vi "ParseSignalConfigCluster.vi"(11 "Signal Channel Config":T1={"Input Mode"=enum."Both Grounded", "Input Connector Shell"=enum."Float", "Input Device"=enum."FET", "Line Rejection Filter"=enum."Off"}) -> (0 "Input Device":bool, 1 "Input Connector Shells":bool, 2 "Input Mode":u16, 3 "Line Frequency\nRejection Filter":u8)   [LabVIEW 2016, in "Instrument.SR7270.lvclass"]
uses:
  Instrument.SR7270.lvclass
  Typedefs/SignalChannelConfig--Cluster.ctl
  Driver/Typedefs/VMODE--enum.ctl
  Driver/SR7270 Drivers.lvclass
  Driver/Typedefs/FLOAT--enum.ctl
  Driver/Typedefs/FET--enum.ctl
  Driver/Typedefs/LF--enum.ctl
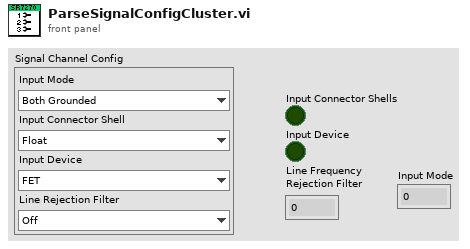
[diagram p1: front panel]
types:
  T1 = typedef "Instrument.SR7270.lvclass/SignalChannelConfig--Cluster.ctl" = cluster{"Input Mode":T2, "Input Connector Shell":T3, "Input Device":T4, "Line Rejection Filter":T5}
  T2 = typedef "SR7270 Drivers.lvclass/VMODE--enum.ctl" = enum16{"Both Grounded", "A input only", "-B input only", "A-B differential"}
  T3 = typedef "SR7270 Drivers.lvclass/FLOAT--enum.ctl" = enum16{"Ground", "Float"}
  T4 = typedef "SR7270 Drivers.lvclass/FET--enum.ctl" = enum16{"Bipolar", "FET"}
  T5 = typedef "SR7270 Drivers.lvclass/LF--enum.ctl" = enum16{"Off", "60 Hz", "120 Hz", "60 & 120 Hz"}
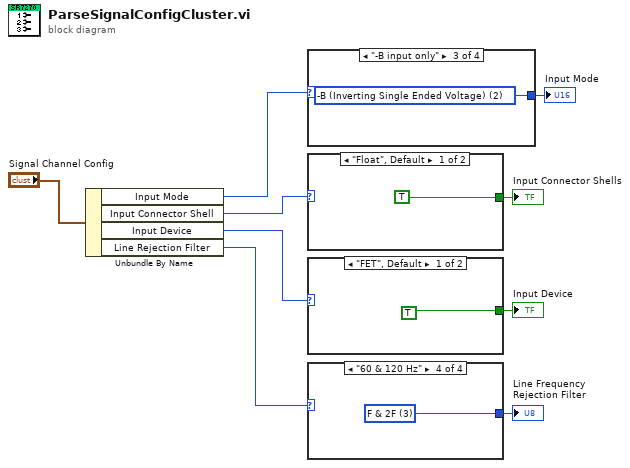
[diagram p0: block diagram]
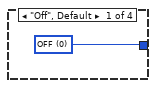
[diagram p2: hidden frame]
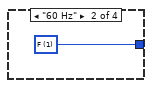
[diagram p3: hidden frame]
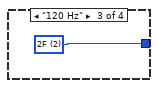
[diagram p4: hidden frame]
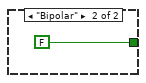
[diagram p5: hidden frame]
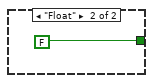
[diagram p6: hidden frame]
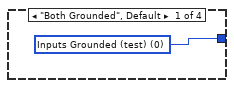
[diagram p7: hidden frame]
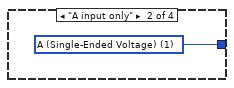
[diagram p8: hidden frame]
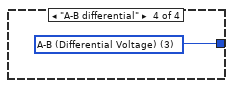
[diagram p9: hidden frame]
diagram:
  n1 = Unbundle By Name("Signal Channel Config") -> ("Input Mode"=w8:T2, "Input Connector Shell"=w7:T3, "Input Device"=w6:T4, "Line Rejection Filter"=w5:T5)
  n2 = case shown="\"-B input only\"" w8 {
    tunnel: [w10 w11 w12 w13] -> w4
    frame "Both Grounded", Default {
      w10 = u16 0 items=["Inputs Grounded (test)", "A (Single-Ended Voltage)", "-B (Inverting Single Ended Voltage)", "A-B (Differential Voltage)"] ("Input Mode")
    }
    frame "A input only" {
      w11 = u16 1 items=["Inputs Grounded (test)", "A (Single-Ended Voltage)", "-B (Inverting Single Ended Voltage)", "A-B (Differential Voltage)"] ("Input Mode")
    }
    frame "-B input only" {
      w12 = u16 2 items=["Inputs Grounded (test)", "A (Single-Ended Voltage)", "-B (Inverting Single Ended Voltage)", "A-B (Differential Voltage)"] ("Input Mode")
    }
    frame "A-B differential" {
      w13 = u16 3 items=["Inputs Grounded (test)", "A (Single-Ended Voltage)", "-B (Inverting Single Ended Voltage)", "A-B (Differential Voltage)"] ("Input Mode")
    }
  }
  "Input Mode" <- w4
  n3 = case shown="\"Float\", Default" w7 {
    tunnel: [TRUE ("Input Connector Shells") FALSE ("Input Connector Shells")] -> w3
    frame "Float", Default {
    }
    frame "Float" {
    }
  }
  "Input Connector Shells" <- w3
  n4 = case shown="\"FET\", Default" w6 {
    tunnel: [TRUE ("Input Device") FALSE ("Input Device")] -> w2
    frame "FET", Default {
    }
    frame "Bipolar" {
    }
  }
  "Input Device" <- w2
  n5 = case shown="\"60 & 120 Hz\"" w5 {
    tunnel: [w18 w19 w20 w21] -> w1
    frame "Off", Default {
      w18 = u8 0 items=["OFF", "F", "2F", "F & 2F"] ("Line Frequency\nRejection Filter")
    }
    frame "60 Hz" {
      w19 = u8 1 items=["OFF", "F", "2F", "F & 2F"] ("Line Frequency\nRejection Filter")
    }
    frame "120 Hz" {
      w20 = u8 2 items=["OFF", "F", "2F", "F & 2F"] ("Line Frequency\nRejection Filter")
    }
    frame "60 & 120 Hz" {
      w21 = u8 3 items=["OFF", "F", "2F", "F & 2F"] ("Line Frequency\nRejection Filter")
    }
  }
  "Line Frequency\nRejection Filter" <- w1
